vi "U04184.vi"(1 "R (Ohm)":dbl=4203.0 format="%.5f") -> (0 "T (K)":dbl=0.29275308045912907 format="%.6f")   [LabVIEW 2018]
panel:
  in  "high range":T1={"ZL"=3.34532592031, "1"=18.2161, "2"=-18.085502, "3"=6.30719, "4"=-1.827232, "5"=0.494402, "6"=-0.125533, "7"=0.027743, "8"=-0.006698, "9"=0.003679, "ZU"=3.44958295882, "10"=0.0} {"10" format="%#_14g"; "ZU" format="%#_12g"; "ZL" format="%#_14g"; "1" format="%#_14g"; "2" format="%#_14g"; "3" format="%#_14g"; "4" format="%#_14g"; "5" format="%#_14g"; "6" format="%#_14g"; "7" format="%#_14g"; "8" format="%#_14g"; "9" format="%#_14g"}
  in  "middle range":T1={"ZL"=3.41973233024, "1"=2.781978, "2"=-3.062546, "3"=1.366584, "4"=-0.553517, "5"=0.208109, "6"=-0.074351, "7"=0.02524, "8"=-0.007465, "9"=0.002348, "ZU"=3.69823716588, "10"=0.0} {"10" format="%#_14g"; "ZU" format="%#_12g"; "ZL" format="%#_14g"; "1" format="%#_14g"; "2" format="%#_14g"; "3" format="%#_14g"; "4" format="%#_14g"; "5" format="%#_14g"; "6" format="%#_14g"; "7" format="%#_14g"; "8" format="%#_14g"; "9" format="%#_14g"}
  out "Z":dbl
  out "k":dbl
  in  "low range":T1={"ZL"=3.62079584778, "1"=0.296224, "2"=-0.382254, "3"=0.199639, "4"=-0.095095, "5"=0.042764, "6"=-0.019139, "7"=0.008222, "8"=-0.003247, "9"=0.001658, "ZU"=4.81728764961, "10"=-0.000563} {"10" format="%#_14g"; "ZU" format="%#_12g"; "ZL" format="%#_14g"; "1" format="%#_14g"; "2" format="%#_14g"; "3" format="%#_14g"; "4" format="%#_14g"; "5" format="%#_14g"; "6" format="%#_14g"; "7" format="%#_14g"; "8" format="%#_14g"; "9" format="%#_14g"}
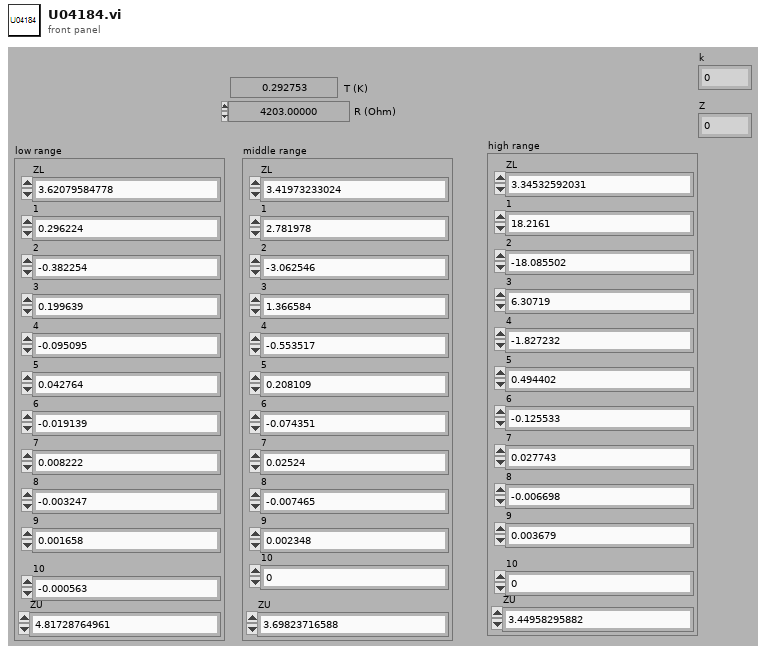
[diagram p1: front panel]
types:
  T1 = cluster{"ZL":dbl, "1":dbl, "2":dbl, "3":dbl, "4":dbl, "5":dbl, "6":dbl, "7":dbl, "8":dbl, "9":dbl, "ZU":dbl, "10":dbl}
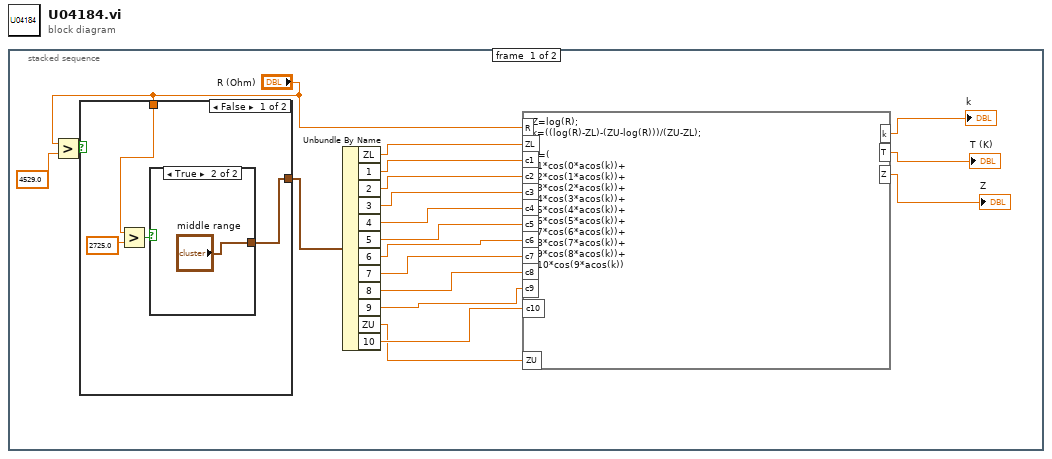
[diagram p0: block diagram]
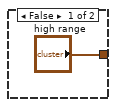
[diagram p2: hidden frame]
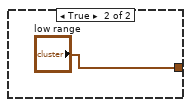
[diagram p3: hidden frame]
diagram:
  n1 = stacked-sequence {
    frame #0 {
      n2 = Greater?(x="R (Ohm)", y=4529.0) -> (0:w6:bool)
      n3 = case shown="False" w6 {
        tunnel: [w23 "low range"] -> w3
        tunnel: "R (Ohm)" -> [w21 _]
        frame False {
          n4 = Greater?(x=w21, y=2725.0) -> (0:w22:bool)
          n5 = case shown="True" w22 {
            tunnel: ["high range" "middle range"] -> w23
            frame False {
            }
            frame True {
            }
          }
        }
        frame True {
        }
      }
      n6 = Unbundle By Name(w3) -> ("ZL"=w9:dbl, "1"=w10:dbl, "2"=w11:dbl, "3"=w12:dbl, "4"=w13:dbl, "5"=w14:dbl, "6"=w15:dbl, "7"=w16:dbl, "8"=w17:dbl, "9"=w18:dbl, "ZU"=w1:dbl, "10"=w2:dbl)
      n7 = formula code="Z=log(R);\nk=((log(R)-ZL)-(ZU-log(R)))/(ZU-ZL);\n\nT=(\nc1*cos(0*acos(k))+\nc2*cos(1*acos(k))+\nc3*cos(2*acos(k))+\nc4*cos(3*acos(k))+\nc5*cos(4*acos(k))+\nc6*cos(5*acos(k))+\nc7*cos(6*acos(k))+\nc8*cos(7*acos(k))+\nc9*cos(8*acos(k))+\nc10*cos(9*acos(k))\n);"("R"="R (Ohm)", "ZL"=w9, "c1"=w10, "c2"=w11, "c3"=w12, "c4"=w13, "c5"=w14, "c6"=w15, "c7"=w16, "c8"=w17, "c9"=w18, "ZU"=w1, "c10"=w2) -> ("T"=→"T (K)":dbl, "k"=→"k":dbl, "Z"=→"Z":dbl)
    }
    frame #1 {
    }
  }
